vi "Handle getAll.vi"(8 "error in (no error)":errorcluster, 11 "Inst.Attocube-3DR in":refnum<class "Inst.Attocube-3DR.lvclass">) -> (0 "error out":errorcluster, 2 "getAll":variant, 3 "Inst.Attocube-3DR out":refnum<class "Inst.Attocube-3DR.lvclass">)   [LabVIEW 2019, in "Inst.Attocube-3DR.lvclass"]
uses:
  Inst.Attocube-3DR.lvclass
  Typedefs/Inst.Attocube-3DR.getAll--Cluster.ctl
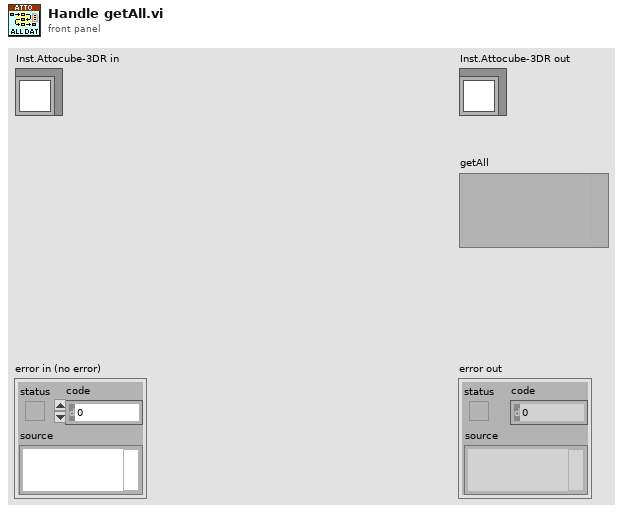
[diagram p1: front panel]
types:
  T1 = typedef "Inst.Attocube-3DR.lvclass/Inst.Attocube-3DR.getAll--Cluster.ctl" = cluster{"Axis 1: Amplitude":dbl, "Axis 1: Capacitance":dbl, "Axis 1: Current Position":dbl, "Axis 1: DCLevel":dbl, "Axis 1: Frequency":dbl, "Axis 1: StepWidth":dbl, "Axis 1: control mode":dbl, "Axis 1: rot. count":dbl, "Axis 1: sp position":dbl, "Axis 1: sp rot. count":dbl, "Axis 1: speed":dbl, "Axis 1: Target GND":bool, "Axis 1: Output":bool, "Axis 1: Single Circle Mode":bool, "Axis 1: moving":bool, "Axis 1: stop detected":bool, "Axis 1:  sensor error":bool, "Axis 1: sensor diconnected":bool, "Axis 1: stop enable":bool, "Axis 2: Current Position":dbl, "Axis 2: DCLevel":dbl, "Axis 2: Frequency":dbl, "Axis 2: StepWidth":dbl, "Axis 2: control mode":dbl, "Axis 2: rot. count":dbl, "Axis 2: sp position":dbl, "Axis 2: sp rot. count":dbl, "Axis 2: speed":dbl, "Axis 2: Capacitance":dbl, "Axis 2: Amplitude":dbl, "Axis 2: Target GND":bool, "Axis 2: Output":bool, "Axis 2: Single Circle Mode":bool, "Axis 2: moving":bool, "Axis 2: stop detected":bool, "Axis 2:  sensor error":bool, "Axis 2: sensor diconnected":bool, "Axis 2: stop enable":bool}
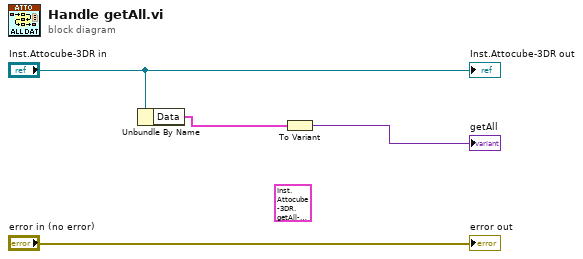
[diagram p0: block diagram]
diagram:
  (unwired) T1 {"Axis 1: Amplitude"=0.0, "Axis 1: Capacitance"=0.0, "Axis 1: Current Position"=0.0, "Axis 1: DCLevel"=0.0, "Axis 1: Frequency"=0.0, "Axis 1: StepWidth"=0.0, "Axis 1: control mode"=0.0, "Axis 1: rot. count"=0.0, "Axis 1: sp position"=0.0, "Axis 1: sp rot. count"=0.0, "Axis 1: speed"=0.0, "Axis 1: Target GND"=FALSE, "Axis 1: Output"=FALSE, "Axis 1: Single Circle Mode"=FALSE, "Axis 1: moving"=FALSE, "Axis 1: stop detected"=FALSE, "Axis 1:  sensor error"=FALSE, "Axis 1: sensor diconnected"=FALSE, "Axis 1: stop enable"=FALSE, "Axis 2: Current Position"=0.0, "Axis 2: DCLevel"=0.0, "Axis 2: Frequency"=0.0, "Axis 2: StepWidth"=0.0, "Axis 2: control mode"=0.0, "Axis 2: rot. count"=0.0, "Axis 2: sp position"=0.0, "Axis 2: sp rot. count"=0.0, "Axis 2: speed"=0.0, "Axis 2: Capacitance"=0.0, "Axis 2: Amplitude"=0.0, "Axis 2: Target GND"=FALSE, "Axis 2: Output"=FALSE, "Axis 2: Single Circle Mode"=FALSE, "Axis 2: moving"=FALSE, "Axis 2: stop detected"=FALSE, "Axis 2:  sensor error"=FALSE, "Axis 2: sensor diconnected"=FALSE, "Axis 2: stop enable"=FALSE} ("getAll")
  n1 = Unbundle By Name("Inst.Attocube-3DR in") -> ("Data"=w2:T1)
  n2 = To Variant(anything=w2) -> (Variant=→"getAll":variant)
  "error out" <- "error in (no error)"
  "Inst.Attocube-3DR out" <- "Inst.Attocube-3DR in"
